vi "ms to Hz.vi"(1 "ms":u32) -> (0 "Numeric":dbl)   [LabVIEW 2019, in "Instrument.DAQ.lvclass"]
uses:
  Instrument.DAQ.lvclass
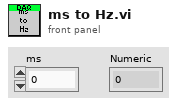
[diagram p1: front panel]
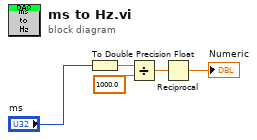
[diagram p0: block diagram]
diagram:
  n1 = To Double Precision Float(number="ms") -> (double precision float=w2:dbl)
  n2 = Divide(x=w2, y=1000.0 ("x")) -> (x/y=w4:dbl)
  n3 = Reciprocal(x=w4) -> (1/x=→"Numeric":dbl)
